vi "mono-grat.vi"(8 "Error In":errorcluster, 10 "Set":bool, 11 "Mono":refnum<vi>) -> (0 "Error Out":errorcluster)   [LabVIEW 2016]
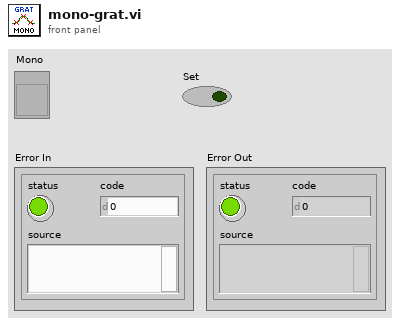
[diagram p1: front panel]
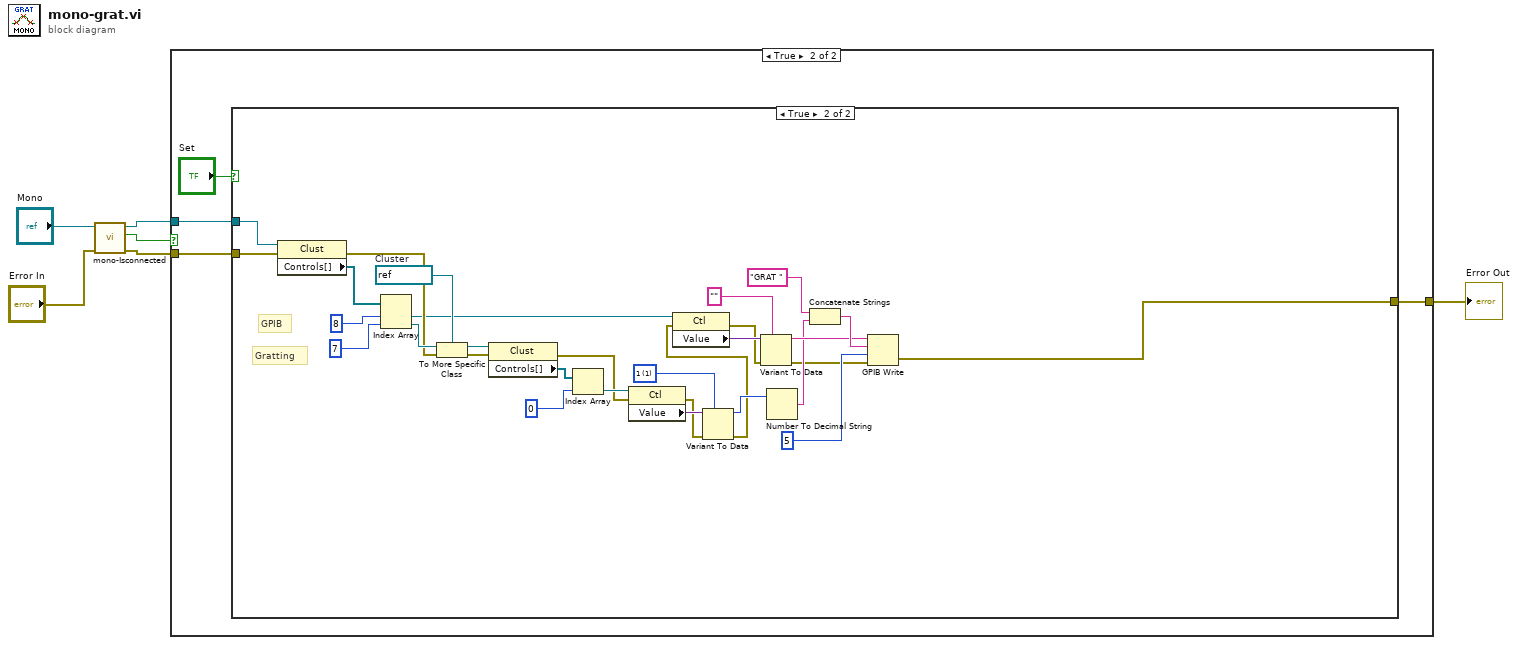
[diagram p0: block diagram]
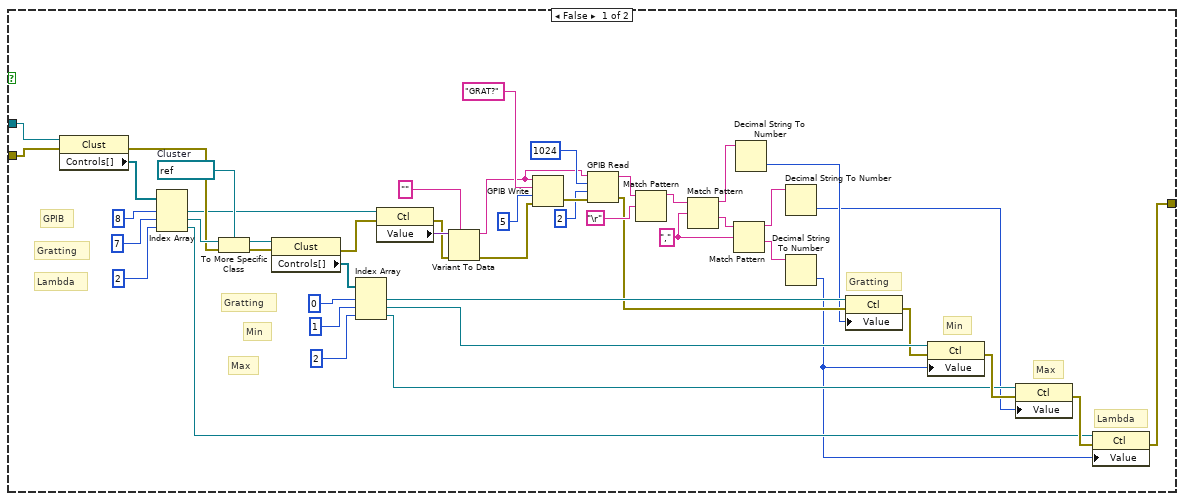
[diagram p3: hidden frame]
diagram:
  n1 = call "mono-Isconnected.vi"("error in (no error)"="Error In", "Monochromator"="Mono") -> ("error out"=w2:errorcluster, "Connected"=w4:bool, "Monochromator out"=w3:refnum<vi>)  [unwired: 7 in]
  n2 = case shown="True" w4 {
    tunnel: [w7 w8] -> w6
    tunnel: w3 -> [_ w10]
    tunnel: w2 -> [w7 w11]
    frame False {
    }
    frame True {
      n3 = case shown="True" "Set" {
        tunnel: w11 -> [w51 w82]
        tunnel: w10 -> [w52 w81]
        tunnel: [w12 w59] -> w8
        frame False {
          w32 = ","
          w55 = refnum<vi> refnum  # Cluster
          # "Lambda"
          # "Max"
          # "Min"
          # "Gratting"
          # "Lambda"
          # "Max"
          # "Gratting"
          # "Min"
          # "Gratting"
          # "GPIB"
          n4 = property class="Clust"(reference=w52, error in=w51) -> (error out=w53:errorcluster, "Controls[]"=w58:refnum<vi>[])  [unwired: 1 out]
          n5 = Index Array(array=w58, index #1=8 ("index"), index #2=7 ("index"), index #3=2 ("index")) -> (element #1=w40:refnum<vi>, element #2=w54:refnum<vi>, element #3=w14:refnum<vi>)
          n6 = To More Specific Class(target class=w55, reference=w54, error in=w53) -> (specific class reference=w48:refnum<vi>, error out=w47:errorcluster)
          n7 = property class="Clust"(reference=w48, error in=w47) -> (error out=w41:errorcluster, "Controls[]"=w50:refnum<vi>[])  [unwired: 1 out]
          n8 = Index Array(array=w50, index #1=0 ("index"), index #2=1 ("index"), index #3=2 ("index")) -> (element #1=w26:refnum<vi>, element #2=w21:refnum<vi>, element #3=w18:refnum<vi>)
          n9 = property class="Ctl"(reference=w40, error in=w41) -> (error out=w38:errorcluster, "Value"=w39:variant)  [unwired: 1 out]
          n10 = Variant To Data(error in=w38, type="", Variant=w39) -> (data=w35:string, error out=w36:errorcluster)
          n11 = GPIB Write(0:w35, 1:"GRAT?" ("data"), 2:i16 5 ("mode (0)"), 3:w36) -> (6:w44:errorcluster)  [unwired: 1 in, 1 out]
          n12 = GPIB Read(0:w35, 1:1024 ("byte count"), 2:i16 2 ("mode (0)"), 3:w44) -> (5:w31:string, 7:w25:errorcluster)  [unwired: 1 in, 1 out]
          n13 = Match Pattern(string=w31, regular expression="\r") -> (before substring=w34:string)  [unwired: 1 in, 3 out]
          n14 = Match Pattern(string=w34, regular expression=w32) -> (before substring=w29:string, after substring=w33:string)  [unwired: 1 in, 2 out]
          n15 = Match Pattern(string=w33, regular expression=w32) -> (before substring=w28:string, after substring=w27:string)  [unwired: 1 in, 2 out]
          n16 = Decimal String To Number(string=w29) -> (number=w24:i32)  [unwired: 2 in, 1 out]
          n17 = Decimal String To Number(string=w28) -> (number=w17:i32)  [unwired: 2 in, 1 out]
          n18 = Decimal String To Number(string=w27) -> (number=w13:i32)  [unwired: 2 in, 1 out]
          n19 = property class="Ctl"(reference=w26, error in=w25, "Value"=w24) -> (error out=w20:errorcluster)  [unwired: 1 out]
          n20 = property class="Ctl"(reference=w21, error in=w20, "Value"=w13) -> (error out=w19:errorcluster)  [unwired: 1 out]
          n21 = property class="Ctl"(reference=w18, error in=w19, "Value"=w17) -> (error out=w15:errorcluster)  [unwired: 1 out]
          n22 = property class="Ctl"(reference=w14, error in=w15, "Value"=w13) -> (error out=w12:errorcluster)  [unwired: 1 out]
        }
        frame True {
          w69 = u8 1 items=["1"=1, "2"=2] ("Number")
          w80 = refnum<vi> refnum  # Cluster
          # "Gratting"
          # "GPIB"
          n23 = property class="Clust"(reference=w81, error in=w82) -> (error out=w78:errorcluster, "Controls[]"=w85:refnum<vi>[])  [unwired: 1 out]
          n24 = Index Array(array=w85, index #1=8 ("index"), index #2=7 ("index")) -> (element #1=w67:refnum<vi>, element #2=w79:refnum<vi>)
          n25 = To More Specific Class(target class=w80, reference=w79, error in=w78) -> (specific class reference=w77:refnum<vi>, error out=w76:errorcluster)
          n26 = property class="Clust"(reference=w77, error in=w76) -> (error out=w72:errorcluster, "Controls[]"=w75:refnum<vi>[])  [unwired: 1 out]
          n27 = Index Array(array=w75, index=0) -> (element=w73:refnum<vi>)
          n28 = property class="Ctl"(reference=w73, error in=w72) -> (error out=w70:errorcluster, "Value"=w71:variant)  [unwired: 1 out]
          n29 = Variant To Data(error in=w70, type=w69, Variant=w71) -> (data=w68:u8, error out=w66:errorcluster)
          n30 = property class="Ctl"(reference=w67, error in=w66) -> (error out=w63:errorcluster, "Value"=w65:variant)  [unwired: 1 out]
          n31 = Variant To Data(error in=w63, type="", Variant=w65) -> (data=w62:string, error out=w60:errorcluster)
          n32 = Number To Decimal String(number=w68) -> (decimal integer string=w61:string)  [unwired: 1 in]
          n33 = Concatenate Strings("GRAT ", w61) -> (w87:string)
          n34 = GPIB Write(0:w62, 1:w87, 2:i16 5 ("mode (0)"), 3:w60) -> (6:w59:errorcluster)  [unwired: 1 in, 1 out]
        }
      }
    }
  }
  "Error Out" <- w6
